vi "Measurement.vi"(4 "Wire in":T1) -> (0 "Classical bit":bool, 1 "Wire out":T1)   [LabVIEW 2016]
uses:
  TypeDefs/Circuit Cluster.ctl
  Classes/GateAbst/GateAbst.lvclass
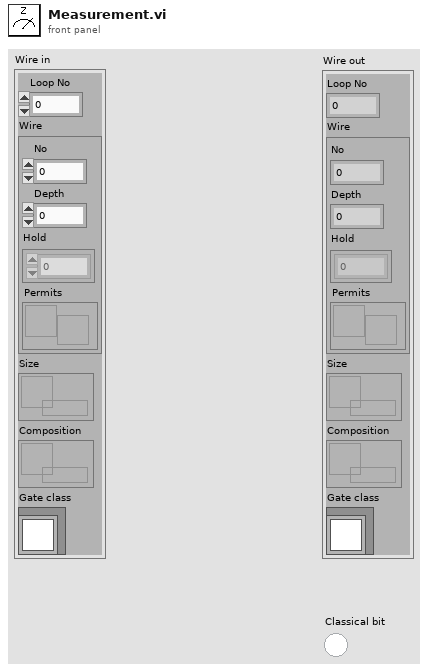
[diagram p1: front panel]
types:
  T1 = typedef "Circuit Cluster.ctl" = cluster{"Loop No":i32, "Wire":cluster{"No":i32, "Depth":i32, "Hold":i32[][], "Permits":refnum<notifier>}, "Size":refnum<queue>, "Composition":refnum<queue>, "Gate class":refnum<class "GateAbst.lvclass">}
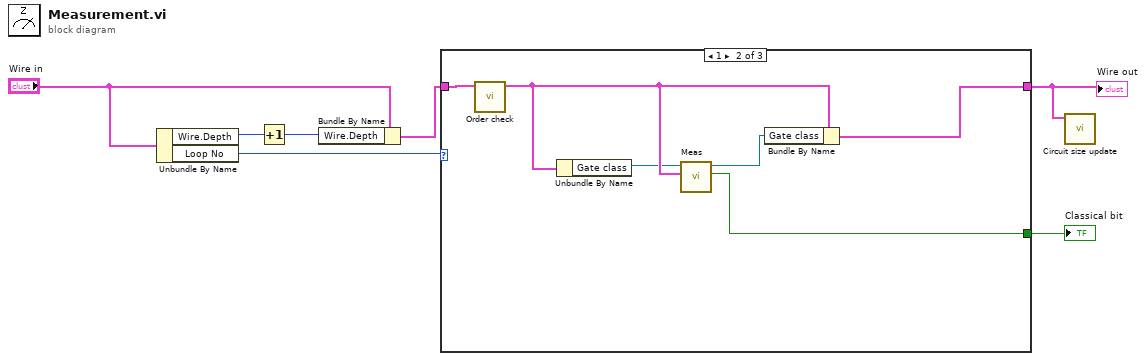
[diagram p0: block diagram]
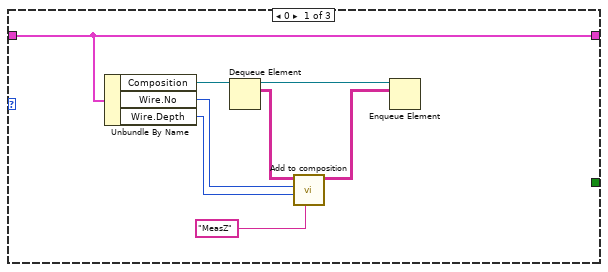
[diagram p2: hidden frame]
diagram:
  n1 = Unbundle By Name("Wire in") -> ("Wire.Depth"=w5:i32, "Loop No"=w1:i32)
  n2 = Increment(x=w5) -> (x+1=w6:i32)
  n3 = Bundle By Name(cluster="Wire in", "Wire.Depth"=w6) -> (w7:T1)
  n4 = case shown="1" w1 {
    tunnel: [w13 w21 w22] -> w3
    tunnel: w7 -> [w13 w19 w22]
    tunnel: [_ w16 _] -> w2
    frame 0 {
      n5 = Unbundle By Name(w13) -> ("Composition"=w14:refnum<queue>, "Wire.No"=w9:i32, "Wire.Depth"=w8:i32)
      n6 = Dequeue Element(queue=w14) -> (queue out=w15:refnum<queue>, element=w10:string[][])  [unwired: 2 in, 2 out]
      n7 = call "Add to composition.vi"("Gate name"="MeasZ", "Wire depth"=w8, "Wire No"=w9, "Composition in"=w10) -> ("Composition out"=w11:string[][])  [unwired: 7 in]
      n8 = Enqueue Element(queue=w15, element=w11) -> ()  [unwired: 2 in, 3 out]
    }
    frame 1 {
      n9 = call "Order check.vi"("Wire in in"=w19) -> ("Wire out"=w18:T1)  [unwired: 10 in]
      n10 = Unbundle By Name(w18) -> ("Gate class"=w17:refnum<class "GateAbst.lvclass">)
      n11 = call-dynamic "Meas.vi"("Wire in"=w18, "GateAbst in"=w17) -> ("Classical bit"=w16:bool, "GateAbst out"=w20:refnum<class "GateAbst.lvclass">)  [unwired: 7 in, 1 out]
      n12 = Bundle By Name(cluster=w18, "Gate class"=w20) -> (w21:T1)
    }
    frame Default {
    }
  }
  "Wire out" <- w3
  "Classical bit" <- w2
  n13 = call "Circuit size update.vi"("Wire in"=w3) -> ()  [unwired: 11 in]
